vi "Sort Frame Array.vi"(11 "Detection Frame In in":T1[](array[typedef]) {"robots_blue"."orientation" format="%+4.3f"; "robots_blue"."y" format="%+4.3f"; "robots_blue"."confidence" format="%4.3f"; "robots_blue"."x" format="%+4.3f"; "robots_yellow"."orientation" format="%+4.3f"; "robots_yellow"."y" format="%+4.3f"; "robots_yellow"."confidence" format="%4.3f"; "robots_yellow"."x" format="%+4.3f"}) -> (3 "Array":T1[](array[typedef]) {"robots_blue"."orientation" format="%+4.3f"; "robots_blue"."y" format="%+4.3f"; "robots_blue"."confidence" format="%4.3f"; "robots_blue"."x" format="%+4.3f"; "robots_yellow"."orientation" format="%+4.3f"; "robots_yellow"."y" format="%+4.3f"; "robots_yellow"."confidence" format="%4.3f"; "robots_yellow"."x" format="%+4.3f"})   [LabVIEW 2017]
uses:
  SSL Detection Frame.ctl
  SSL Detection Robot.ctl
  <vilib>/Analysis/Matrix/Datatypes/RealMatrix.ctl
  SSL Detection Ball.ctl
  <vilib>/Analysis/Matrix/NI_Matrix.lvlib
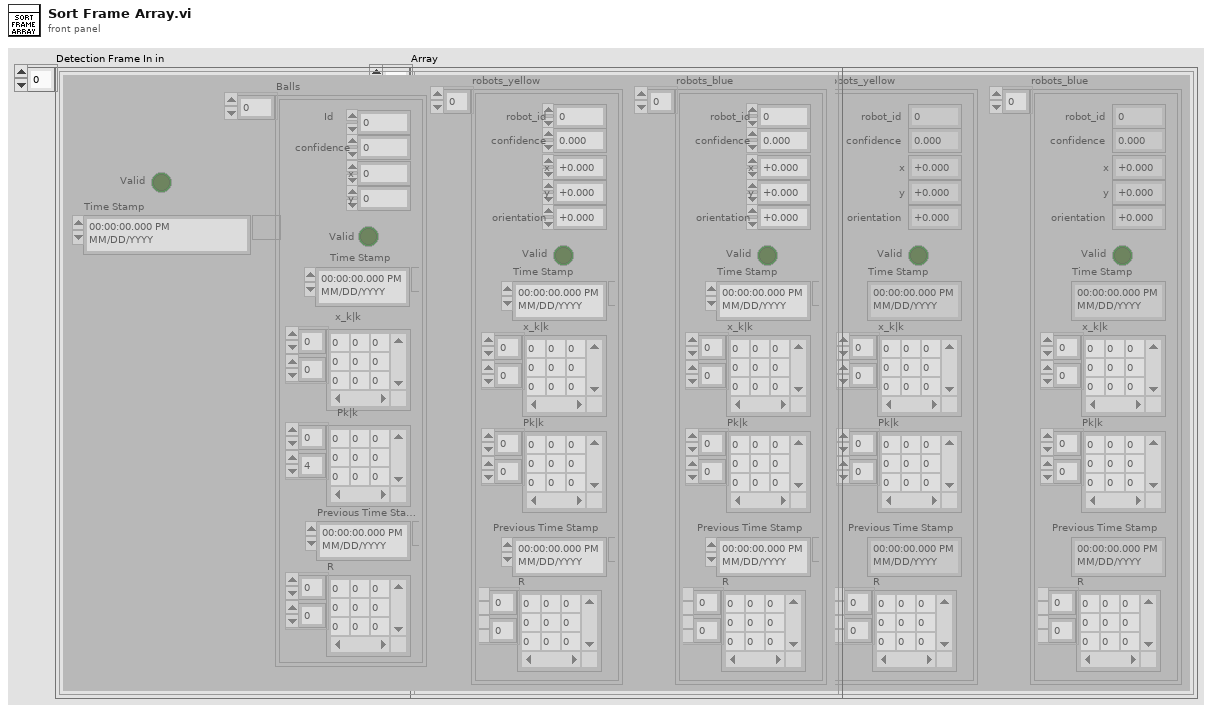
[diagram p1: front panel]
types:
  T1 = typedef "SSL Detection Frame.ctl" = cluster{"robots_yellow":T2[], "robots_blue":T2[], "Valid":bool, "Time Stamp":timestamp, "Balls":T4[]}
  T2 = typedef "SSL Detection Robot.ctl" = cluster{"x":sgl, "robot_id":u32, "confidence":sgl, "y":sgl, "orientation":sgl, "Valid":bool, "Time Stamp":timestamp, "x_k|k":T3, "Pk|k":T3, "Previous Time Stamp":timestamp, "R":T3}
  T3 = typedef "NI_Matrix.lvlib/RealMatrix.ctl" = dbl[][]
  T4 = typedef "SSL Detection Ball.ctl" = cluster{"x":sgl, "confidence":sgl, "y":sgl, "Valid":bool, "Time Stamp":timestamp, "x_k|k":T3, "Pk|k":T3, "Id":u32, "Previous Time Stamp":timestamp, "R":T3}
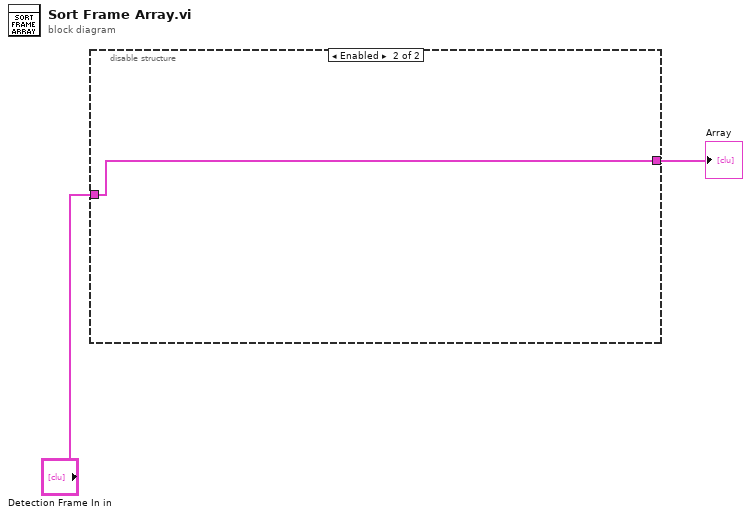
[diagram p0: block diagram]
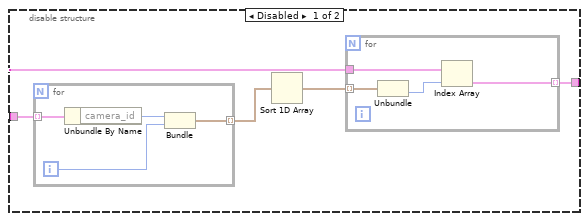
[diagram p2: hidden frame]
diagram:
  n1 = disable-structure shown="Enabled" {
    disable-tunnel: [w6 w15] -> w2
    disable-tunnel: "Detection Frame In in" -> [w5 w15]
    frame Disabled {
      n2 = for {
        tunnel: w5 -> [w11] mode=indexing
        tunnel: [w12] -> w3 mode=indexing
        i -> [w13]
        n3 = Unbundle By Name(w11) -> ("camera_id"=w14:u32)
        n4 = Bundle("camera_id"=w14, w13) -> (w12:cluster{"camera_id":u32, i32})  [unwired: 1 in]
      }
      n5 = Sort 1D Array(array=w3) -> (sorted array=w4:cluster{"camera_id":u32, i32}[])
      n6 = for {
        tunnel: w4 -> [w9] mode=indexing
        tunnel: w5 -> [w10]
        tunnel: [w7] -> w6 mode=indexing
        n7 = Unbundle(w9) -> (w8:i32)  [unwired: 1 out]
        n8 = Index Array(array=w10, index=w8) -> (element=w7:T1)
      }
    }
    frame Enabled {
    }
  }
  "Array" <- w2
